vi "replaceAmountToken.vi"(8 "error in (no error)":errorcluster, 10 "Query In":string, 11 "UserEditableAmount in":refnum<class "UserEditableAmount.lvclass">) -> (0 "error out":errorcluster, 2 "Query Out":string, 3 "UserEditableAmount out":refnum<class "UserEditableAmount.lvclass">)   [LabVIEW 2018, in "UserEditableAmount.lvclass"]
uses:
  UserEditableAmount.lvclass
  UserEditableAmount.lvclass/UserEditableAmount.ctl
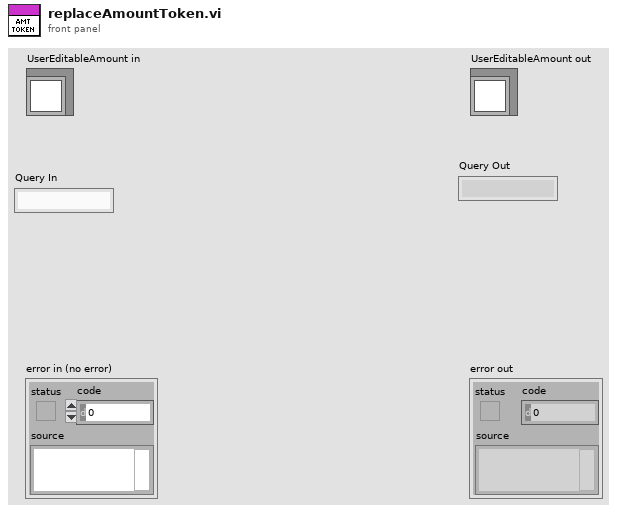
[diagram p1: front panel]
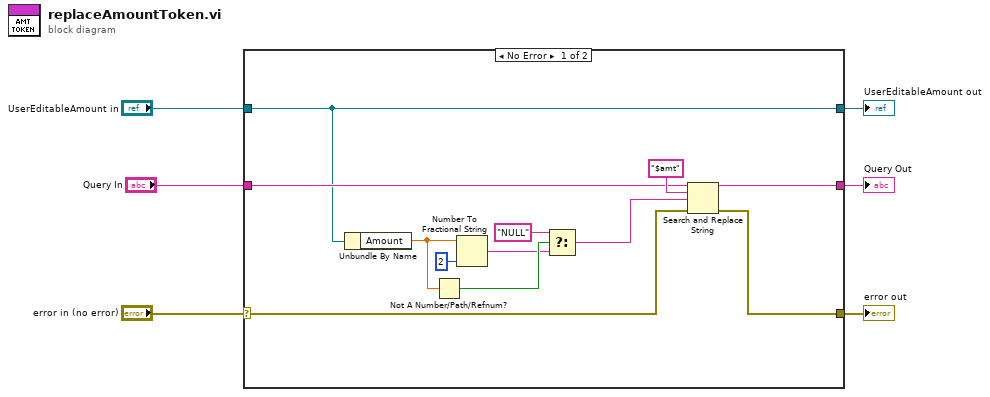
[diagram p0: block diagram]
diagram:
  n1 = case shown="No Error" "error in (no error)" {
    selector: "error in (no error)" -> [w12 w21]
    tunnel: [w11 w21] -> w5
    tunnel: [w8 w20] -> w3
    tunnel: "UserEditableAmount in" -> [w8 w20]
    tunnel: [w10 w19] -> w2
    tunnel: "Query In" -> [w9 w19]
    frame No Error {
      n2 = Unbundle By Name(w8) -> ("Amount"=w7:dbl)
      n3 = Not A Number/Path/Refnum?(number/path/refnum=w7) -> (NaN/Path/Refnum?=w16:bool)
      n4 = Number To Fractional String(number=w7, precision (6)=i16 2) -> (F-format string=w15:string)  [unwired: 2 in]
      n5 = Select(t="NULL", s=w16, f=w15) -> (s? t:f=w13:string)
      n6 = Search and Replace String(input string=w9, search string="$amt", replace string=w13, error in=w12) -> (result string=w10:string, error out=w11:errorcluster)  [unwired: 4 in, 2 out]
    }
    frame Error {
    }
  }
  "error out" <- w5
  "UserEditableAmount out" <- w3
  "Query Out" <- w2
